vi "CAN发车速 - 副本.vi"() -> ()   [LabVIEW 2020]
uses:
  ZLG_CAN/ZLG_CAN.lvlib
panel:
  out "数组":u8[](array[numeric])
  in  "Stop":bool
  in  "周期(ms)":u32=10 min=1 format="%d ms"
  in  "帧格式":enum16{"数据帧", "远程帧"}(ring)
  in  "帧类型":enum8{"标准帧", "扩展帧"}(ring)
  in  "ID":u32=745 format="0x%x"
  in  "波特率":u32(ring)=11 items=["5Kbps", "10Kbps", "20Kbps", "40Kbps", "50Kbps", "80Kbps", "100Kbps", "125Kbps", "200Kbps", "250Kbps", "400Kbps", "500Kbps", "666Kbps", "800Kbps", "1000Kbps"]
  in  "CAN 通道":u32(ring) items=["0", "1"]
  in  "索引":u32(ring) items=["0", "1", "2", "3", "4", "5", "6", "7", "8"]
  in  "设备类型":u32(ring)=3 items=["PCI5121"=1, "PCI9810"=2, "USBCAN1"=3, "USBCAN2"=4, "PCI9820"=5, "PCI5110"=7, "PC104CAN"=11, "CANETUDP"=12, "PCI9840B"=14, "PC104C2"=15, "PCI9820I"=16, "CANETTCP"=17, "PCIE9221"=24, "PCI5010U"=19, "USBCAN_E_U"=20, "USBCAN_2E_U"=21, "PCI5020U"=22, "PCIE9120I"=27, "PCIE9110I"=28, "PCIE9140I"=29]
  in  "Stop":bool
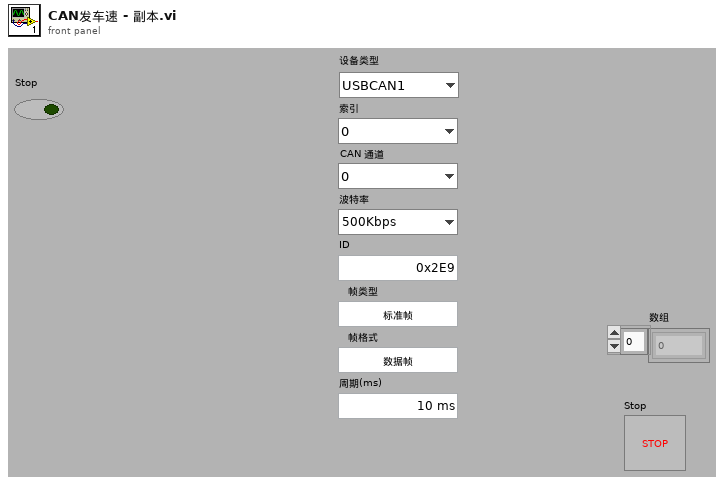
[diagram p1: front panel]
types:
  T1 = typedef "ZLG_CAN.lvlib/Start_CAN (Reply Payload)--cluster.ctl" = cluster{"Success":bool, "Start_CAN_error":errorcluster}
  T2 = cluster{u8, u8, "y":u8, "y":u8, "y":u8, "y":u8, "y":u8, "y":u8}
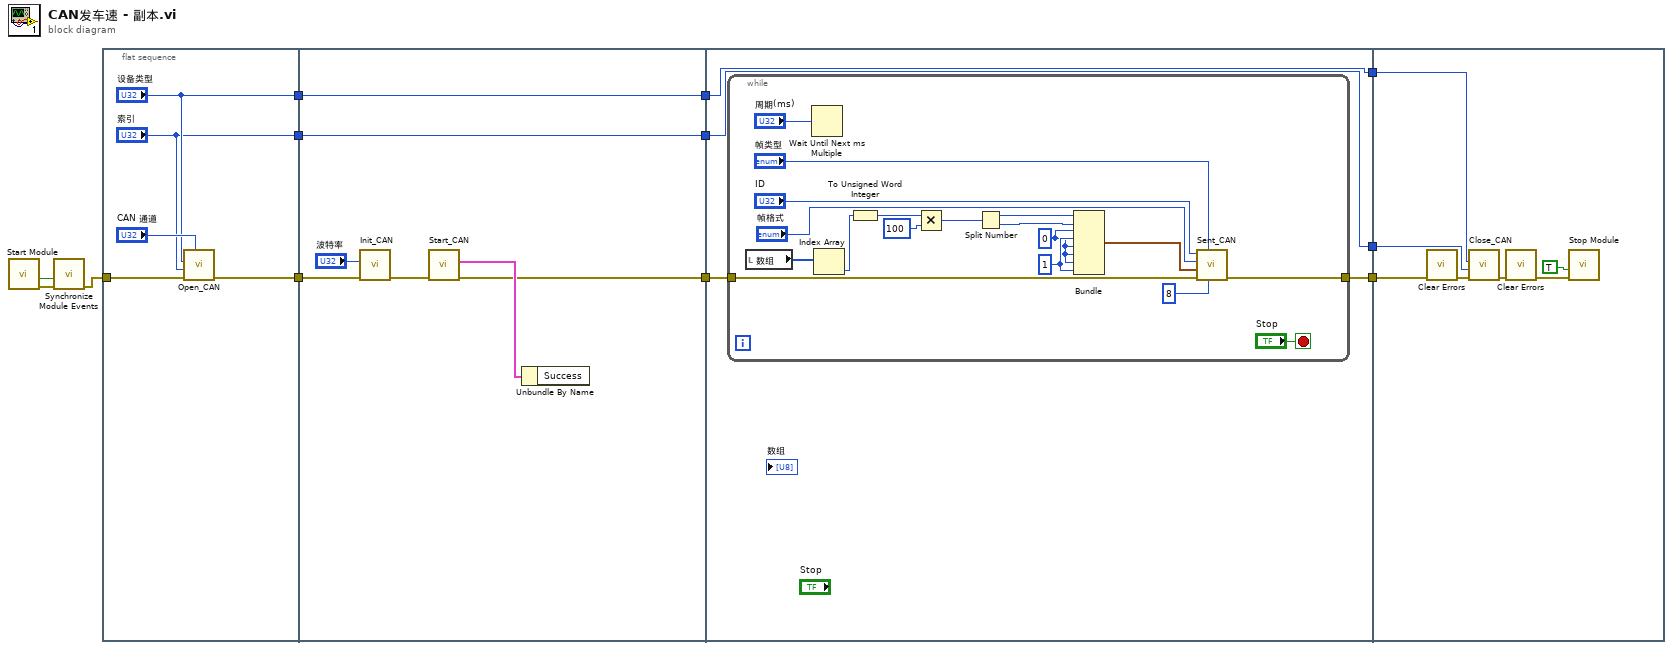
[diagram p0: block diagram]
diagram:
  n1 = call "Start Module.vi"() -> ("error out"=w3:errorcluster, "Wait for Event Sync?"=w2:bool)  [unwired: 8 in, 2 out]
  n2 = call "Synchronize Module Events.vi"("error in (no error)"=w3, "Wait for Event Sync?"=w2) -> ("error out"=w1:errorcluster)  [unwired: 9 in]
  n3 = flat-sequence {
    tunnel: ["索引"] -> w6
    tunnel: ["设备类型"] -> w5
    tunnel: [w15] -> w4
    tunnel: w1 -> [w13]
    tunnel: [w23] -> w12
    tunnel: [w20] -> w10
    tunnel: [w21] -> w8
    tunnel: w6 -> [w21]
    tunnel: w5 -> [w20]
    tunnel: w4 -> [w19]
    tunnel: w12 -> [w28]
    tunnel: [w27] -> w11
    tunnel: w10 -> [w26]
    tunnel: [w26] -> w9
    tunnel: w8 -> [w25]
    tunnel: [w25] -> w7
    tunnel: w11 -> [w53]
    tunnel: w9 -> [w52]
    tunnel: w7 -> [w51]
    frame #0 {
      n4 = call "Open_CAN.vi"("CAN 通道"="CAN 通道", "error in (no error)"=w13, "索引"="索引", "设备类型"="设备类型") -> ("error out"=w15:errorcluster)  [unwired: 7 in]
    }
    frame #1 {
      n5 = call "Init_CAN.vi"("error in (no error)"=w19, "波特率"="波特率") -> ("error out"=w22:errorcluster)  [unwired: 9 in]
      n6 = call "Start_CAN.vi"("error in (no error)"=w22) -> ("error out"=w23:errorcluster, "Reply Payload"=w24:T1)  [unwired: 8 in, 1 out]
      n7 = Unbundle By Name(w24) -> ()  [unwired: 1 out]
    }
    frame #2 {
      n8 = while {
        tunnel: w28 -> [w46]
        tunnel: [w45] -> w27
        stop <- "Stop" stop-if-true
        w41 = u8 1 ("y")
        w33 = u8 0 ("y")
        n9 = local read "数组"() -> (w29:u8[])
        n10 = Wait Until Next ms Multiple(millisecond multiple="周期(ms)") -> ()  [unwired: 1 out]
        n11 = Index Array(array=w29) -> (element=w32:u8)  [unwired: 1 in]
        n12 = To Unsigned Word Integer(number=w32) -> (unsigned 16bit integer=w43:u16)
        n13 = Multiply(x=w43, y=u16 100) -> (x*y=w42:u16)
        n14 = Split Number(x=w42) -> (hi(x)=w31:u8, lo(x)=w30:u8)
        n15 = Bundle(w31, w30, "y"=w33, "y"=w41, "y"=w33, "y"=w33, "y"=w33, "y"=w41) -> (w40:T2)  [unwired: 1 in]
        n16 = call "Sent_CAN.vi"("帧长度"=u8 8, "帧类型"="帧类型", "error in (no error)"=w46, "帧数据"=w40, "帧格式"="帧格式", "ID"="ID") -> ("error out"=w45:errorcluster)  [unwired: 5 in]
      }
    }
    frame #3 {
      n17 = call <vilib>:"Clear Errors.vi"("error in (no error)"=w53) -> ("error out"=w47:errorcluster)  [unwired: 5 in, 1 out]
      n18 = call "Close_CAN.vi"("error in (no error)"=w47, "索引"=w51, "设备类型"=w52) -> ("error out"=w50:errorcluster)  [unwired: 8 in]
      n19 = call <vilib>:"Clear Errors.vi"("error in (no error)"=w50) -> ("error out"=w48:errorcluster)  [unwired: 5 in, 1 out]
      n20 = call "Stop Module.vi"("error in (no error)"=w48, "Wait for Module to Stop? (F)"=TRUE) -> ()  [unwired: 9 in, 1 out]
    }
  }
